vi "Query Trigger Delay.vi"(8 "error in (no error)":errorcluster, 11 "VISA resource name":refnum<visa-resource-name>) -> (0 "error out":errorcluster, 2 "delay (s)":dbl, 3 "VISA resource name out":refnum<visa-resource-name>)   [LabVIEW 2019, in "Pulse Rider PG-1000.lvlib"]
doc: "Query the trigger output delay in s"
uses:
  <instrlib>/LV_PulseRiderPG1000/Pulse Rider PG-1000.lvlib
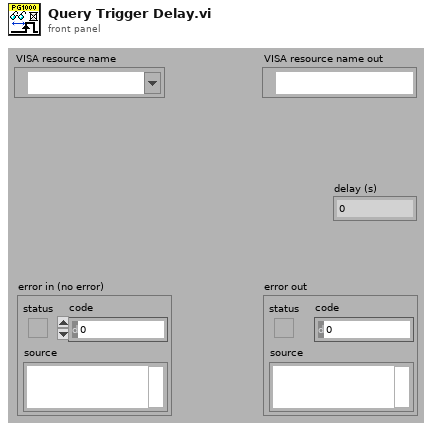
[diagram p1: front panel]
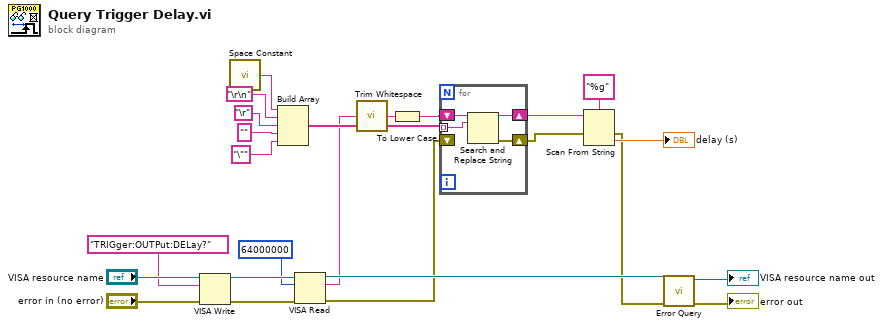
[diagram p0: block diagram]
diagram:
  n1 = VISA Write(VISA resource name="VISA resource name", write buffer="TRIGger:OUTPut:DELay?", error in (no error)="error in (no error)") -> (VISA resource name out=w20:refnum<visa-resource-name>, error out=w19:errorcluster)  [unwired: 1 out]
  n2 = call <vilib>:"Space Constant.vi"() -> ("String"=w15:string)
  n3 = Build Array(w15, "\r\n", "\r", "", "\"") -> (w10:string[])
  n4 = VISA Read(VISA resource name=w20, byte count=u32 64000000, error in (no error)=w19) -> (VISA resource name out=w17:refnum<visa-resource-name>, read buffer=w8:string, error out=w2:errorcluster)  [unwired: 1 out]
  n5 = call <vilib>:"Trim Whitespace.vi"("string"=w8) -> ("trimmed string"=w9:string)  [unwired: 1 in]
  n6 = To Lower Case(string=w9) -> (all lower case string=w7:string)
  n7 = for {
    tunnel: w10 -> [w26] mode=indexing
    shift-right: [w28] -> w6
    shift-left: w7 -> [w27]
    shift-right: [w25] -> w3
    shift-left: w2 -> [_]
    n8 = Search and Replace String(input string=w27, search string=w26) -> (result string=w28:string, error out=w25:errorcluster)  [unwired: 6 in, 2 out]
  }
  n9 = Scan From String(format string="%g", input string=w6, error in=w3) -> (error out=w1:errorcluster, output 1=→"delay (s)":dbl)  [unwired: 2 in, 2 out]
  n10 = call <instrlib>:"Error Query.vi"("error in (no error)"=w1, "VISA resource name"=w17) -> ("error out"=→"error out":errorcluster, "VISA resource name out"=→"VISA resource name out":refnum<visa-resource-name>)  [unwired: 6 in, 2 out]
